vi "Create Arrows.vi"(7 "Height Padding":dbl format="%#_13g", 10 "Drawing Info Parent":T1, 11 "Drawing Info Child":T2) -> (3 "Arrows":cluster{dbl, dbl}[](array[cluster]))   [LabVIEW 2025]
panel:
  in  "Arrow Length":dbl=5.0 format="%#_13g"
  in  "Arrow Width":dbl=5.0 format="%#_13g"
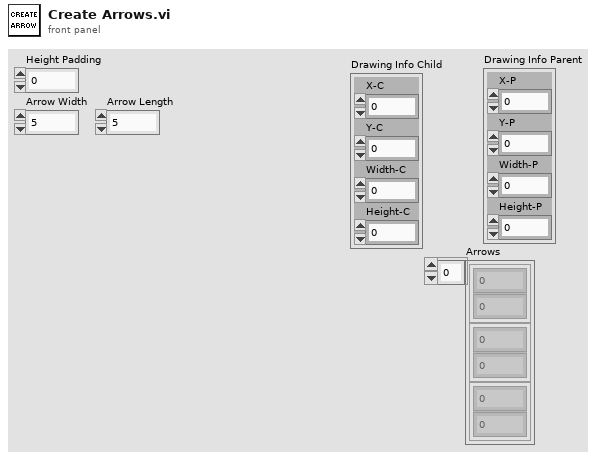
[diagram p1: front panel]
types:
  T1 = cluster{"X-P":dbl, "Y-P":dbl, "Width-P":dbl, "Height-P":dbl}
  T2 = cluster{"X-C":dbl, "Y-C":dbl, "Width-C":dbl, "Height-C":dbl}
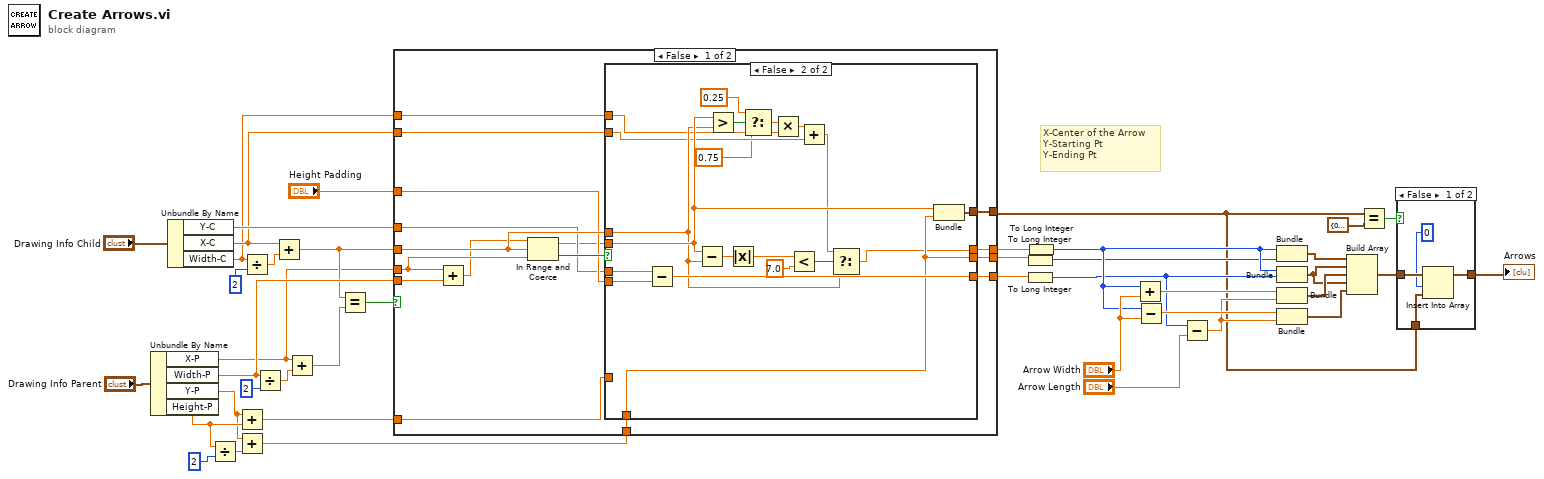
[diagram p0: block diagram]
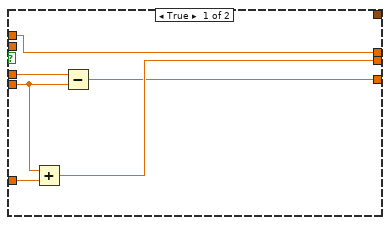
[diagram p3: hidden frame]
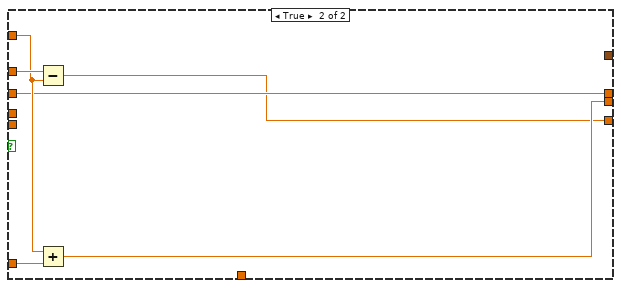
[diagram p4: hidden frame]
diagram:
  # "X-Center of the Arrow\nY-Starting Pt\nY-Ending Pt"
  n1 = Unbundle By Name("Drawing Info Parent") -> ("X-P"=w4:dbl, "Width-P"=w31:dbl, "Y-P"=w11:dbl, "Height-P"=w14:dbl)
  n2 = Unbundle By Name("Drawing Info Child") -> ("Y-C"=w34:dbl, "X-C"=w2:dbl, "Width-C"=w1:dbl)
  n3 = Divide(x=w14, y=2) -> (x/y=w12:dbl)
  n4 = Add(x=w11, y=w14) -> (x+y=w33:dbl)
  n5 = Add(x=w11, y=w12) -> (x+y=w10:dbl)
  n6 = Divide(x=w1, y=2) -> (x/y=w39:dbl)
  n7 = Divide(x=w31, y=2) -> (x/y=w37:dbl)
  n8 = Add(x=w2, y=w39) -> (x+y=w21:dbl)
  n9 = Add(x=w4, y=w37) -> (x+y=w9:dbl)
  n10 = Equal?(x=w21, y=w9) -> (x = y?=w36:bool)
  n11 = case shown="False" w36 {
    tunnel: w34 -> [w49 w89]
    tunnel: w33 -> [w51 w88]
    tunnel: "Height Padding" -> [w52 w87]
    tunnel: w21 -> [w54 w86]
    tunnel: w4 -> [w57 _]
    tunnel: w31 -> [w56 _]
    tunnel: [w53 w86] -> w20
    tunnel: [w50 w85] -> w18
    tunnel: [w48 w84] -> w16
    tunnel: w10 -> [w46 _]
    tunnel: [w45 _] -> w3
    tunnel: w2 -> [w42 _]
    tunnel: w1 -> [w43 _]
    frame False {
      n12 = Add(x=w57, y=w56) -> (x+y=w47:dbl)
      n13 = In Range and Coerce(upper limit=w47, x=w54, lower limit=w57) -> (coerced(x)=w44:dbl, In Range?=w55:bool)
      n14 = case shown="False" w55 {
        tunnel: w54 -> [w60 w72]
        tunnel: [w60 w71] -> w53
        tunnel: w52 -> [w58 w81]
        tunnel: w51 -> [w63 _]
        tunnel: [w62 w79] -> w50
        tunnel: w49 -> [w61 w83]
        tunnel: [w59 w82] -> w48
        tunnel: w46 -> [_ w79]
        tunnel: [_ w80] -> w45
        tunnel: w44 -> [_ w73]
        tunnel: w43 -> [_ w67]
        tunnel: w42 -> [_ w66]
        frame True {
          n15 = Add(x=w58, y=w63) -> (x+y=w62:dbl)
          n16 = Subtract(x=w61, y=w58) -> (x-y=w59:dbl)
        }
        frame False {
          n17 = Subtract(x=w83, y=w81) -> (x-y=w82:dbl)
          n18 = Subtract(x=w73, y=w72) -> (x-y=w78:dbl)
          n19 = Greater?(x=w73, y=w72) -> (0:w74:bool)
          n20 = Absolute Value(x=w78) -> (abs(x)=w75:dbl)
          n21 = Select(t=0.25, s=w74, f=0.75) -> (s? t:f=w70:dbl)
          n22 = Multiply(x=w70, y=w67) -> (x*y=w69:dbl)
          n23 = Less?(x=w75, y=7.0) -> (x < y?=w76:bool)
          n24 = Add(x=w69, y=w66) -> (x+y=w68:dbl)
          n25 = Select(t=w68, s=w76, f=w72) -> (s? t:f=w71:dbl)
          n26 = Bundle("X-P"=w73, w79) -> (w80:cluster{"X-P":dbl, dbl})  [unwired: 1 in]
        }
      }
    }
    frame True {
      n27 = Subtract(x=w89, y=w87) -> (x-y=w84:dbl)
      n28 = Add(x=w87, y=w88) -> (x+y=w85:dbl)
    }
  }
  n29 = To Long Integer(number=w18) -> (32bit integer=w17:i32)
  n30 = To Long Integer(number=w16) -> (32bit integer=w15:i32)
  n31 = To Long Integer(number=w20) -> (32bit integer=w19:i32)
  n32 = Add(x=w19, y="Arrow Width") -> (x+y=w24:dbl)
  n33 = Subtract(x=w19, y="Arrow Width") -> (x-y=w25:dbl)
  n34 = Subtract(x=w15, y="Arrow Length") -> (x-y=w22:dbl)
  n35 = Bundle(w19, w17) -> (w30:cluster{i32, i32})  [unwired: 1 in]
  n36 = Bundle(w19, w15) -> (w28:cluster{i32, i32})  [unwired: 1 in]
  n37 = Bundle(w24, w22) -> (w29:cluster{dbl, dbl})  [unwired: 1 in]
  n38 = Bundle(w25, w22) -> (w27:cluster{dbl, dbl})  [unwired: 1 in]
  n39 = Build Array(w30, w28, w29, w28, w27) -> (w8:cluster{dbl, dbl}[])
  n40 = Equal?(x=w3, y=cluster{dbl, dbl} {0.0, 0.0}) -> (x = y?=w7:bool)
  n41 = case shown="False" w7 {
    tunnel: w8 -> [w93 w94]
    tunnel: w3 -> [w91 _]
    tunnel: [w92 w94] -> w5
    frame False {
      n42 = Insert Into Array(array=w93, index=0, new element=w91) -> (w92:cluster{dbl, dbl}[])
    }
    frame True {
    }
  }
  "Arrows" <- w5
